vi "ShowWindowARGB.vi"(8 "error in (no error)":errorcluster, 10 "Window Name":string, 11 "ARGB Image":refnum<data-value>) -> (0 "error out":errorcluster, 3 "ARGB Image (duplicate)":refnum<data-value>)   [LabVIEW 2020, in "g_ar_toolkit.image.lvlib"]
uses:
  g_ar_toolkit.image.lvlib
  g_ar_toolkit.common/Module Path.vi
  <vilib>/Utility/error.llb/Error Cluster From Error Code.vi
  df490a54-c425-41e5-8765-b6fcf549c24a.vi
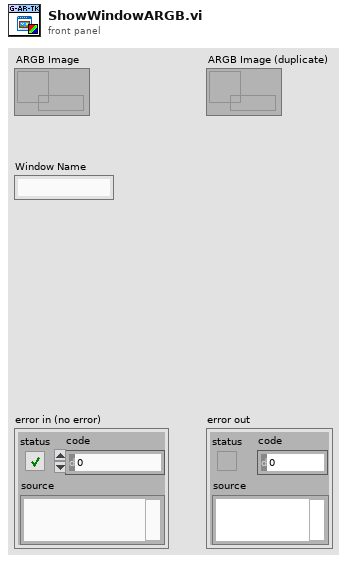
[diagram p1: front panel]
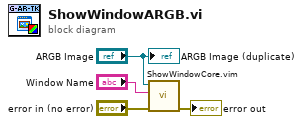
[diagram p0: block diagram]
diagram:
  n1 = call "ShowWindowCore.vim"("error in (no error)"="error in (no error)", "Window Name"="Window Name", "Img"="ARGB Image") -> ("error out"=→"error out":errorcluster)  [unwired: 8 in]
  "ARGB Image (duplicate)" <- "ARGB Image"
